vi "H5Fmount.vi"(5 "HDF5 Property List Ref":T1, 6 "error in (no error)":errorcluster, 7 "HDF5 Child Ref":T1, 8 "Group":string, 9 "HDF5 Ref":T1) -> (0 "error out":errorcluster, 3 "HDF5 Ref out":T1)   [LabVIEW 2017]
doc: "Mounts a file."
uses:
  <vilib>/UPVI/lvhdf5/library.llb/HDF5 Ref.ctl
  <vilib>/UPVI/lvhdf5/hdf5.dll
panel:
  # "LVHDF5 Toolkit\nCopyright (c) 2005-2013 by Jason D. Sommerville\nCopyright (c) 2014 by UPVI, LLC.\n\nThis use and distribution of this file is governed by the terms found in \nLICENSE.txt distributed with this toolkit and installed at\n <user.lib>\\_lvhdf5\\LICENSE.txt"
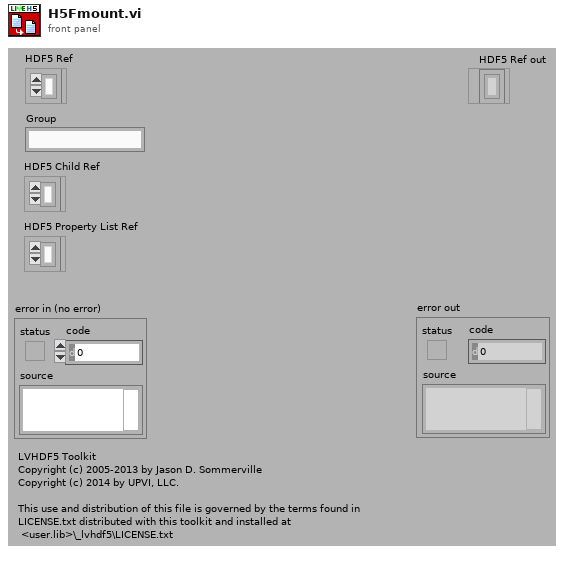
[diagram p1: front panel]
types:
  T1 = typedef "HDF5 Ref.ctl" = refnum<k1>
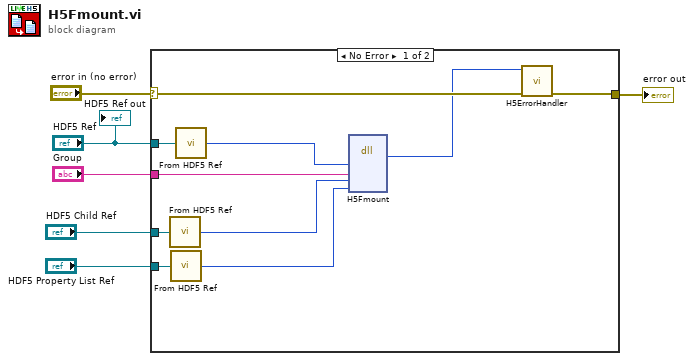
[diagram p0: block diagram]
diagram:
  n1 = case shown="No Error" "error in (no error)" {
    selector: "error in (no error)" -> [w16 w17]
    tunnel: [w15 w17] -> w5
    tunnel: "HDF5 Ref" -> [w12 _]
    tunnel: "Group" -> [w13 _]
    tunnel: "HDF5 Child Ref" -> [w10 _]
    tunnel: "HDF5 Property List Ref" -> [w8 _]
    frame No Error {
      n2 = call <vilib>:"From HDF5 Ref.vi"("HDF5 Ref"=w10) -> ("I32"=w9:i32)
      n3 = call <vilib>:"From HDF5 Ref.vi"("HDF5 Ref"=w8) -> ("I32"=w7:i32)
      n4 = call <vilib>:"From HDF5 Ref.vi"("HDF5 Ref"=w12) -> ("I32"=w11:i32)
      n5 = dll-call lib="C:/Program Files/National Instruments/LabVIEW 2017/vi.lib/UPVI/lvhdf5/hdf5.dll" fn="H5Fmount"("loc_id"=w11, "name"=w13, "child_id"=w9, "plist_id"=w7) -> (w14:i32)  [unwired: 7 in, 2 out]
      n6 = call <vilib>:"H5ErrorHandler.vi"("error in (no error)"=w16, "herr_t"=w14) -> ("error out"=w15:errorcluster)  [unwired: 3 in, 4 out]
    }
    frame Error {
    }
  }
  "error out" <- w5
  "HDF5 Ref out" <- "HDF5 Ref"
